vi "JSON_extract_Data_2 (SubVI).vi"(8 "data":T1, 11 "cluster in":string) -> (2 "id":u8, 3 "data":T1)   [LabVIEW 2015]
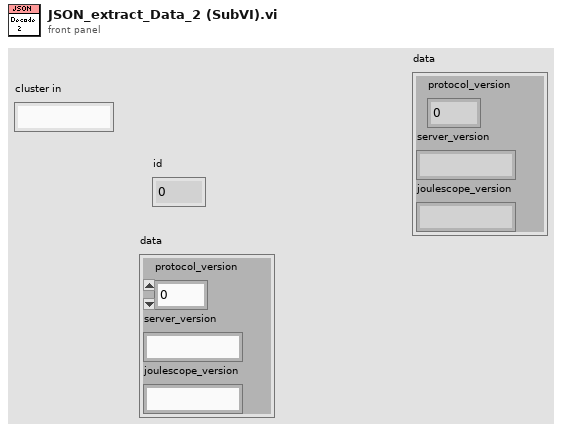
[diagram p1: front panel]
types:
  T1 = cluster{"protocol_version":i32, "server_version":string, "joulescope_version":string}
  T2 = cluster{"type":string, "phase":string, "id":u8, "status":i32, "status_msg":string, "device":string, "data":cluster{"protocol_version":i32, "server_version":string, "joulescope_version":string}}
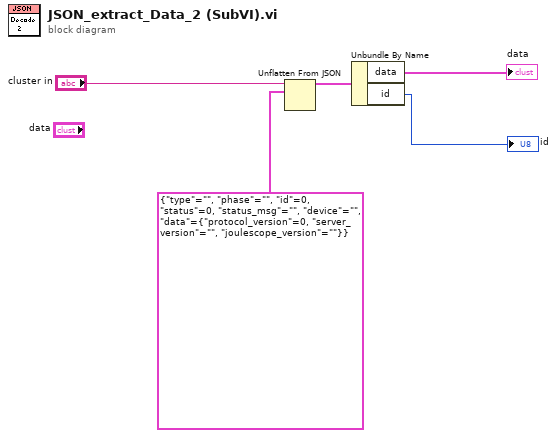
[diagram p0: block diagram]
diagram:
  n1 = Unflatten From JSON(JSON string="cluster in", type and defaults=T2 {"type"="", "phase"="", "id"=0, "status"=0, "status_msg"="", "device"="", "data"={"protocol_version"=0, "server_version"="", "joulescope_version"=""}}) -> (value=w5:T2)  [unwired: 5 in, 1 out]
  n2 = Unbundle By Name(w5) -> ("data"=→"data":T1, "id"=→"id":u8)
